vi "error.vi"(8 "error in (no error)":errorcluster, 11 "Output Value":i32) -> (0 "error out":errorcluster)   [LabVIEW 2014, in "AvaSpec.lvlib" / "Avantes Spectrometer Functions.lvlib"]
uses:
  Avantes Spectrometer Functions.lvlib
  AvaSpec.lvlib
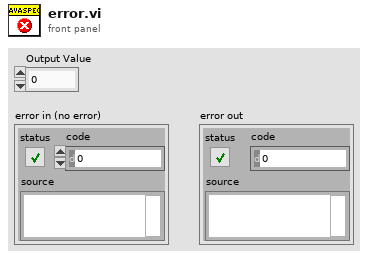
[diagram p1: front panel]
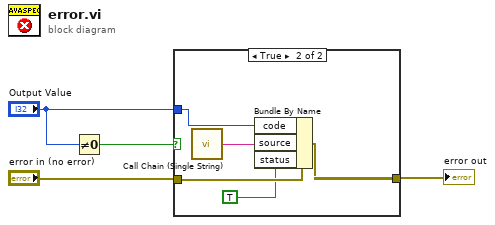
[diagram p0: block diagram]
diagram:
  n1 = Not Equal To 0?(x="Output Value") -> (x != 0?=w4:bool)
  n2 = case shown="True" w4 {
    tunnel: "error in (no error)" -> [w5 w10]
    tunnel: [w5 w9] -> w2
    tunnel: "Output Value" -> [_ w8]
    frame False {
    }
    frame True {
      n3 = call "Call Chain (Single String).vi"() -> ("Call Chain"=w7:string)
      n4 = Bundle By Name(cluster=w10, "code"=w8, "source"=w7, "status"=TRUE) -> (w9:errorcluster)
    }
  }
  "error out" <- w2
